vi "New.vi"(11 "Msg Output in":refnum<class "Msg Output.lvclass">) -> (0 "Error out":errorcluster, 3 "Msg Output out":refnum<class "Msg Output.lvclass">)   [LabVIEW 2020, in "jettl.lvlib" / "Msg Output.lvclass"]
uses:
  Msg Output.lvclass
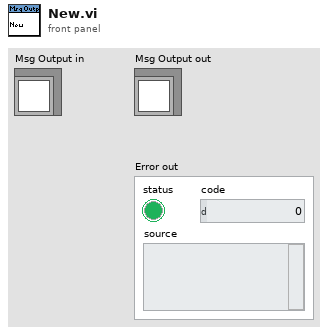
[diagram p1: front panel]
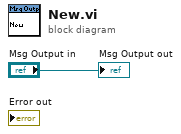
[diagram p0: block diagram]
diagram:
  "Msg Output out" <- "Msg Output in"
